vi "Create Engine Group from Channel Array.vi"(7 "Group Name":string, 8 "error in (no error)":errorcluster, 9 "Type":T3(ring)=enum."Input/Read", 10 "Item Names":string[](array[string]), 11 "Device Item Ref in":T1 format="%.0x") -> (0 "error out":errorcluster, 2 "output cluster":T2 {"VS Refs" format="%.0x"}, 3 "Device Item Ref out":T1=18446744073709551615 format="%.0x")   [LabVIEW 2015, in "Modbus Master System Explorer.lvlib"]
uses:
  Modbus Master System Explorer.lvlib
  <vilib>/NI Veristand/Custom Device API/Custom Device Item Ref.ctl
  <vilib>/NI Veristand/Custom Device Tools/Custom Device Utility Library/NI VeriStand - Search for Item by Name.vi
  <vilib>/NI VeriStand/Custom Device API/Custom Device API.lvlib
  <vilib>/NI VeriStand/Custom Device Tools/Custom Device Utility Library/Custom Device Utility Library.lvlib
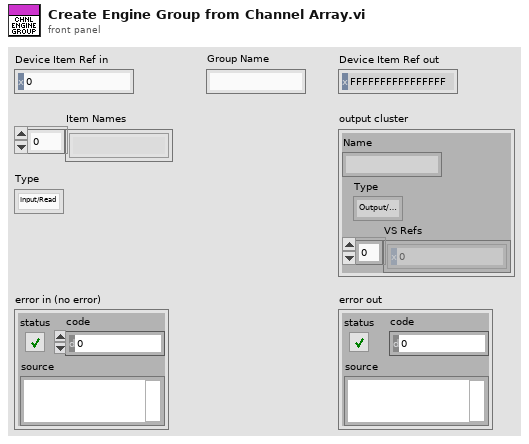
[diagram p1: front panel]
types:
  T1 = typedef "Custom Device API.lvlib/Custom Device Item Ref.ctl" = u64
  T2 = cluster{"Name":string, "Type":enum16{"Output/Write", "Input/Read", "Input/ReadWrite"}, "VS Refs":T1[]}
  T3 = enum16{"Output/Write", "Input/Read", "Input/ReadWrite"}
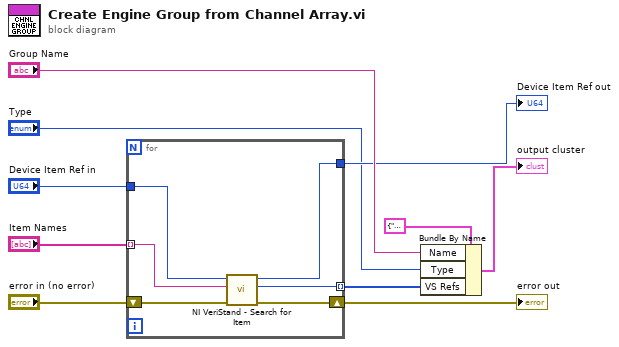
[diagram p0: block diagram]
diagram:
  n1 = for {
    tunnel: "Item Names" -> [w16] mode=indexing
    tunnel: "Device Item Ref in" -> [w15]
    tunnel: [w14] -> w5
    shift-right: [w12] -> w1
    shift-left: "error in (no error)" -> [w13]
    tunnel: [w11] -> w3 mode=indexing
    n2 = call-poly <vilib>:"NI VeriStand - Search for Item.vi"("error in"=w13, "Item Name"=w16, "Section Ref in"=w15) -> ("error out"=w12:errorcluster, "Item Ref"=w11:T1, "Section Ref out"=w14:T1)  [unwired: 5 in, 1 out]
  }
  "Device Item Ref out" <- w5
  "error out" <- w1
  n3 = Bundle By Name(cluster=T2 {"Name"="", "Type"=enum."Input/Read", "VS Refs"=[]} ("Group"), "Name"="Group Name", "Type"="Type", "VS Refs"=w3) -> (→"output cluster":T2)
